vi "Fetch Multi Eval Meas Modulation Detected Allocation Results.vi"(8 "error in (no error)":errorcluster, 10 "Instance (1)":T2=1, 11 "VISA resource name":refnum<visa-resource-name>) -> (0 "error out":errorcluster, 1 "Detected Allocation":T1, 2 "Reliability":i32, 3 "VISA resource name out":refnum<visa-resource-name>)   [LabVIEW 2015, in "Rohde&Schwarz CMXP NR FR2 Measurement.lvlib"]
doc: "Returns the detected allocation for the measured slot.\n\nAttribute:\nRSCMXPNRFR2M_ATTR_FETCH_MULTI_EVAL_MEASUREMENT_MODULATION_DETECTED_ALLOCATION_RESULTS\n\nRemote-control command:\nFETCh:NRMMw:MEAS<i>:MEValuation:MODulation:DALLocation?"
uses:
  <instrlib>/Rohde&Schwarz CMXP NR FR2 Measurement/Rohde&Schwarz CMXP NR FR2 Measurement.lvlib
  <instrlib>/Rohde&Schwarz CMXP NR FR2 Measurement/Private/_Instance.ctl
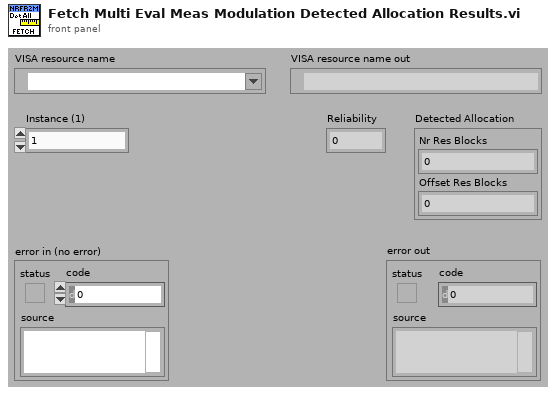
[diagram p1: front panel]
types:
  T1 = cluster{"Nr Res Blocks":i32, "Offset Res Blocks":i32}
  T2 = typedef "Rohde&Schwarz CMXP NR FR2 Measurement.lvlib/_Instance.ctl" = i32
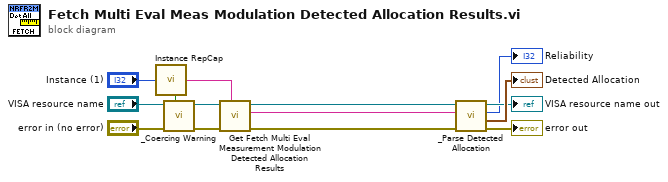
[diagram p0: block diagram]
diagram:
  n1 = call <instrlib>:"Instance RepCap.vi"("Instance In"="Instance (1)") -> ("In Range?"=w3:bool, "RepCap Identifier Out"=w14:string)  [unwired: 1 in]
  n2 = call <instrlib>:"_Coercing Warning.vi"("In Range?"=w3, "error in (no error)"="error in (no error)", "VISA resource name"="VISA resource name") -> ("error out"=w4:errorcluster, "VISA resource name out"=w5:refnum<visa-resource-name>)  [unwired: 7 in]
  n3 = call "Get Fetch Multi Eval Measurement Modulation Detected Allocation Results"("Repeated Capabilities"=w14, "error in (no error)"=w4, "instrument handle"=w5) -> ("error out"=w11:errorcluster, "Fetch Multi Eval Measurement Modulation Detected Allocation Results"=w13:string, "instrument handle out"=w10:refnum<visa-resource-name>)  [unwired: 6 in]
  n4 = call <instrlib>:"_Parse Detected Allocation.vi"("error in (no error)"=w11, "Input String"=w13, "VISA resource name"=w10) -> ("error out"=→"error out":errorcluster, "Detected Allocation"=→"Detected Allocation":T1, "Reliability"=→"Reliability":i32, "VISA resource name out"=→"VISA resource name out":refnum<visa-resource-name>)  [unwired: 5 in]
